vi "Shutdown Processes.vi"(8 "error in (no error)":errorcluster, 11 "Assembler in":refnum<class "Assembler.lvclass">) -> (0 "error out":errorcluster, 3 "Assembler out":refnum<class "Assembler.lvclass">)   [LabVIEW 2019, in "TimingDRV Engine.lvlib" / "Assembler.lvclass"]
uses:
  Assembler.lvclass
  C:/Users/XEnderMD/Desktop/CD Project Tools/Source/Engine/Parent Classes/Process/Process.lvclass
  Parent Classes/Process/Process.lvclass/Process.ctl
  Parent Classes/Process/Process.lvclass
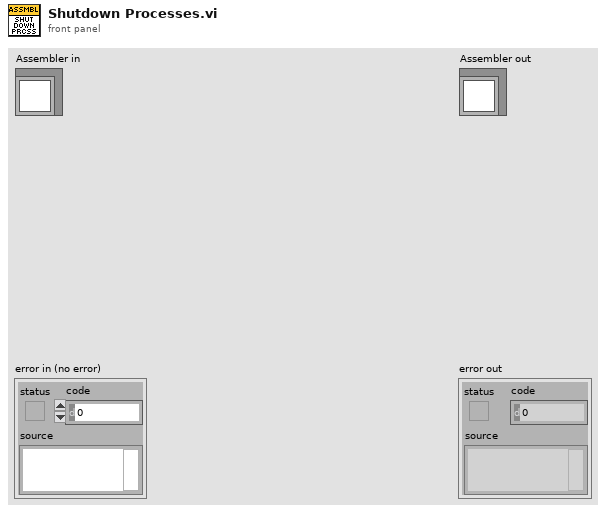
[diagram p1: front panel]
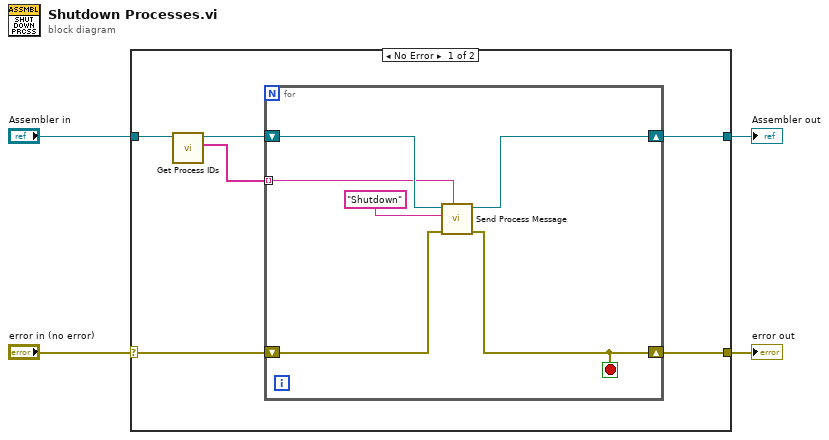
[diagram p0: block diagram]
diagram:
  n1 = case shown="No Error" "error in (no error)" {
    selector: "error in (no error)" -> [w7 w18]
    tunnel: [w6 w18] -> w3
    tunnel: [w5 w17] -> w1
    tunnel: "Assembler in" -> [w10 w17]
    frame No Error {
      n2 = call "Get Process IDs.vi"("Process in"=w10) -> ("Process IDs"=w8:string[], "Process out"=w9:refnum<class "Assembler.lvclass">)  [unwired: 9 in]
      n3 = for {
        shift-right: [w14] -> w5
        shift-left: w9 -> [w16]
        tunnel: w8 -> [w15] mode=indexing
        shift-right: [w11] -> w6
        shift-left: w7 -> [w12]
        stop <- w11 stop-if-true
        n4 = call "Send Process Message.vi"("Process ID"=w15, "error in (no error)"=w12, "Command"="Shutdown", "Process in"=w16) -> ("error out"=w11:errorcluster, "Process out"=w14:refnum<class "Assembler.lvclass">)  [unwired: 6 in]
      }
    }
    frame Error {
    }
  }
  "error out" <- w3
  "Assembler out" <- w1
